vi "StateHapticEngine.vi"(0 "Master State In":T1(ring)) -> ()   [LabVIEW 2020]
doc: "Manages the haptic feedback on the driver and manipulator joysticks."
uses:
  GlobalDriverStationData.vi
  GlobalAutonomous.vi
  GlobalDriverStationCommands.vi
  GRNF_Joystick.vi
  GlobalDrivebase.vi
  GlobalGripper.vi
  GlobalArm.vi
panel:
  in  "setpoint vibration length":u32=1000
  in  "Develop New Haptic":bool
  in  "Duty Cycle (%)":dbl=100.0
  in  "Amplitude":dbl=1.0
  in  "Period (s)":dbl=10.0
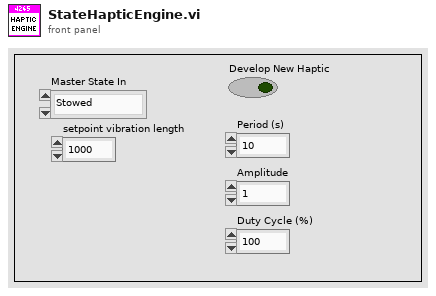
[diagram p1: front panel]
types:
  T1 = enum16{"Stowed", "Balancing", "Scoring", "Hoppering", "Ground", "Shelf"}
  T2 = enum16{"None", "Development", "Longpress Buttons", "End Effector"}
  T3 = typedef "WPI_JoystickDevRef.ctl" = cluster{"Device":T4}
  T4 = typedef "WPI_JoystickDeviceEnum.ctl" = enum16{"USB 0", "USB 1", "USB 2", "USB 3", "USB 4", "USB 5"}
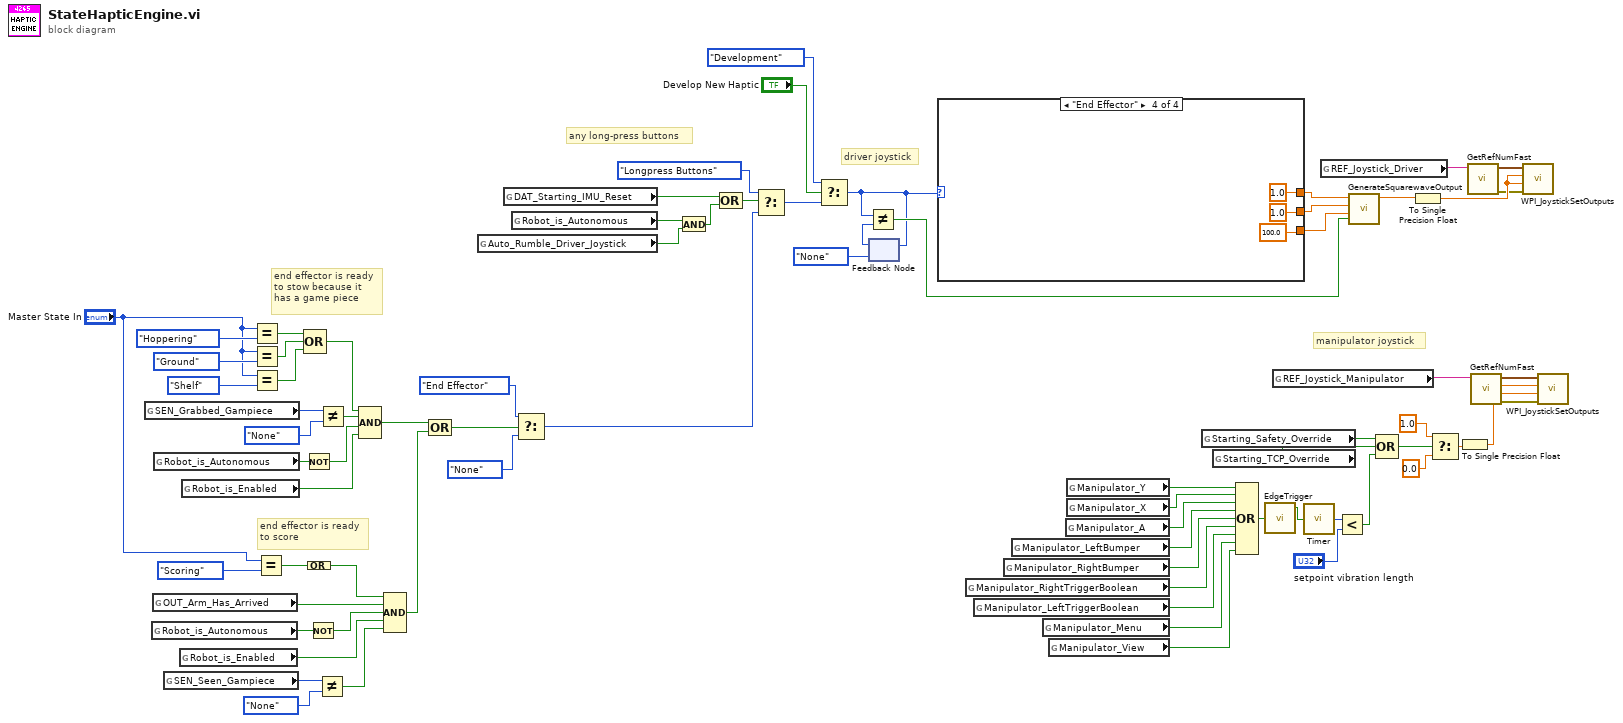
[diagram p0: block diagram]
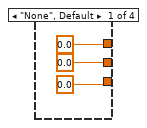
[diagram p2: hidden frame]
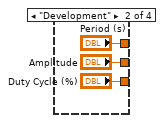
[diagram p3: hidden frame]
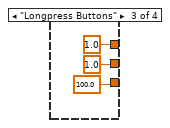
[diagram p4: hidden frame]
diagram:
  # "end effector is ready\nto score"
  # "end effector is ready\nto stow because it\nhas a game piece"
  # "any long-press buttons"
  # "manipulator joystick"
  # "driver joystick"
  n1 = global read "GlobalGripper.vi" "SEN_Grabbed_Gampiece"() -> (w46:enum16{"None", "Cube", "Cone"})
  n2 = global read "GlobalDriverStationData.vi" "Robot_is_Autonomous"() -> (w27:bool)
  n3 = global read "GlobalArm.vi" "OUT_Arm_Has_Arrived"() -> (w18:bool)
  n4 = global read "GlobalDriverStationData.vi" "Robot_is_Autonomous"() -> (w43:bool)
  n5 = global read "GlobalGripper.vi" "SEN_Seen_Gampiece"() -> (w17:enum16{"None", "Cube", "Cone"})
  n6 = global read "GlobalDriverStationData.vi" "Robot_is_Enabled"() -> (w25:bool)
  n7 = global read "GlobalDriverStationData.vi" "Robot_is_Enabled"() -> (w40:bool)
  n8 = Equal?(x="Master State In", y=T1."Hoppering") -> (x = y?=w38:bool)
  n9 = Equal?(x="Master State In", y=T1."Ground") -> (x = y?=w35:bool)
  n10 = Equal?(x="Master State In", y=T1."Shelf") -> (x = y?=w34:bool)
  n11 = Equal?(x="Master State In", y=T1."Scoring") -> (x = y?=w23:bool)
  n12 = Compound Arithmetic op=OR(w38, w35, w34) -> (w33:bool)
  n13 = Not(x=w43) -> (.not. x?=w42:bool)
  n14 = Compound Arithmetic op=OR(w23) -> (w22:bool)
  n15 = Not(x=w27) -> (.not. x?=w26:bool)
  n16 = Not Equal?(x=w17, y=enum16{"None", "Cube", "Cone"}."None") -> (x != y?=w15:bool)
  n17 = Not Equal?(x=w46, y=enum16{"None", "Cube", "Cone"}."None") -> (x != y?=w44:bool)
  n18 = Compound Arithmetic op=AND(w33, w44, w42, w40) -> (w28:bool)
  n19 = Compound Arithmetic op=AND(w22, w18, w26, w25, w15) -> (w21:bool)
  n20 = Compound Arithmetic op=OR(w28, w21) -> (w20:bool)
  n21 = global read "GlobalAutonomous.vi" "Auto_Rumble_Driver_Joystick"() -> (w64:bool)
  n22 = global read "GlobalDrivebase.vi" "DAT_Starting_IMU_Reset"() -> (w47:bool)
  n23 = global read "GlobalDriverStationData.vi" "Robot_is_Autonomous"() -> (w52:bool)
  n24 = Select(t=T2."End Effector", s=w20, f=T2."None") -> (s? t:f=w41:T2)
  n25 = And(x=w52, y=w64) -> (x .and. y?=w63:bool)
  n26 = Compound Arithmetic op=OR(w47, w63) -> (w61:bool)
  n27 = Select(t=T2."Longpress Buttons", s=w61, f=w41) -> (s? t:f=w50:T2)
  n28 = Select(t=T2."Development", s="Develop New Haptic", f=w50) -> (s? t:f=w56:T2)
  n29 = feedback-in #1(w56) -> ()
  n30 = feedback #1(T2."None") -> (w59:T2)
  n31 = Not Equal?(x=w56, y=w59) -> (x != y?=w58:bool)
  n32 = case shown="\"End Effector\"" w56 {
    tunnel: [0.0 ("Period (s)") "Period (s)" 1.0 ("Period (s)") 1.0 ("Period (s)")] -> w55
    tunnel: [0.0 ("Amplitude") "Amplitude" 1.0 ("Amplitude") 1.0 ("Amplitude")] -> w54
    tunnel: [0.0 ("Duty Cycle (%)") "Duty Cycle (%)" 100.0 ("Duty Cycle (%)") 100.0 ("Duty Cycle (%)")] -> w53
    frame "None", Default {
    }
    frame "Development" {
    }
    frame "Longpress Buttons" {
    }
    frame "End Effector" {
    }
  }
  n33 = global read "GlobalDriverStationCommands.vi" "Manipulator_RightTriggerBoolean"() -> (w9:bool)
  n34 = global read "GlobalDriverStationCommands.vi" "Manipulator_LeftTriggerBoolean"() -> (w8:bool)
  n35 = global read "GlobalDriverStationCommands.vi" "Manipulator_RightBumper"() -> (w10:bool)
  n36 = global read "GlobalDriverStationCommands.vi" "Manipulator_LeftBumper"() -> (w11:bool)
  n37 = global read "GlobalDriverStationCommands.vi" "Manipulator_Menu"() -> (w7:bool)
  n38 = global read "GlobalDriverStationCommands.vi" "Manipulator_View"() -> (w6:bool)
  n39 = global read "GlobalDriverStationCommands.vi" "Manipulator_A"() -> (w12:bool)
  n40 = global read "GlobalDriverStationCommands.vi" "Manipulator_Y"() -> (w14:bool)
  n41 = global read "GlobalDriverStationCommands.vi" "Manipulator_X"() -> (w13:bool)
  n42 = global read "GlobalDriverStationData.vi" "Starting_Safety_Override"() -> (w65:bool)
  n43 = global read "GlobalDriverStationData.vi" "Starting_TCP_Override"() -> (w51:bool)
  n44 = Compound Arithmetic op=OR(w14, w13, w12, w11, w10, w9, w8, w7, w6) -> (w5:bool)
  n45 = call "EdgeTrigger.vi"("Input Signal"=w5) -> ("Rising Edge Trigger"=w4:bool)  [unwired: 2 out]
  n46 = global read "GlobalDriverStationCommands.vi" "REF_Joystick_Manipulator"() -> (w49:string)
  n47 = call "Timer.vi"("Reset Timer"=w4) -> ("Time (ms)"=w3:u32)
  n48 = global read "GlobalDriverStationCommands.vi" "REF_Joystick_Driver"() -> (w48:string)
  n49 = Less?(x=w3, y="setpoint vibration length") -> (x < y?=w2:bool)
  n50 = call "GenerateSquarewaveOutput.vi"("Init"=w58, "Duty Cycle (%)"=w53, "Amplitude"=w54, "Period (s)"=w55) -> ("Square Wave Ouput"=w62:dbl)  [unwired: 7 in]
  n51 = Compound Arithmetic op=OR(w65, w51, w2) -> (w70:bool)
  n52 = To Single Precision Float(number=w62) -> (single precision float=w75:sgl)
  n53 = Select(t=1.0, s=w70, f=0.0) -> (s? t:f=w72:dbl)
  n54 = To Single Precision Float(number=w72) -> (single precision float=w71:sgl)
  n55 = call-poly "GetRefNumFast.vi"("RefNum Name"=w48) -> ("Error"=w68:errorcluster, "Device Reference"=w69:T3)  [unwired: 5 in]
  n56 = call-poly "GetRefNumFast.vi"("RefNum Name"=w49) -> ("Error"=w67:errorcluster, "Device Reference"=w66:T3)  [unwired: 5 in]
  n57 = call <vilib>:"WPI_JoystickSetOutputs.vi"("error in (no error)"=w68, "Right Rumble"=w75, "Left Rumble"=w75, "JoystickDevRef"=w69) -> ()  [unwired: 6 in, 2 out]
  n58 = call <vilib>:"WPI_JoystickSetOutputs.vi"("error in (no error)"=w67, "Right Rumble"=w71, "Left Rumble"=w71, "JoystickDevRef"=w66) -> ()  [unwired: 6 in, 2 out]
